vi "Open Form.vi"(8 "error in (no error)":errorcluster, 9 "Caller Name":T1, 10 "Form Config":refnum<class "Form Model Configuration.lvclass">, 11 "Form Server in":refnum<class "Form Server.lvclass">) -> (0 "error out":errorcluster, 3 "Form Server out":refnum<class "Form Server.lvclass">)   [LabVIEW 2020, in "Form Server.lvlib" / "Form Server.lvclass"]
uses:
  Form Server.lvclass
  C:/Program Files (x86)/National Instruments/LabVIEW 2020/vi.lib/ActorFramework/Actor/Actor.lvclass
  Forms Model/Form Model Configuration/Form Model Configuration Class/Form Model Configuration.lvclass
  Autoclose manager/Form ID.ctl
  Form Server.lvclass/Form Server.ctl
  Form Server Configuration/Form Server Configuration.lvclass/Form Server Configuration.ctl
  Forms Model/Form Model Actor/Form Model.lvclass
  Autoclose manager/Open Close Logic.lvclass
  <vilib>/ActorFramework/Actor/Actor.lvclass
  Form Server Configuration/Form Server Configuration.lvclass
  Form Server Interfaces.lvlib
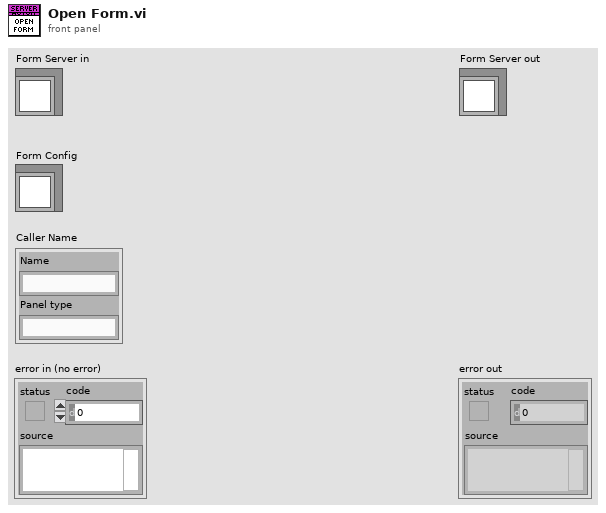
[diagram p1: front panel]
types:
  T1 = typedef "Form Server Interfaces.lvlib/Form ID.ctl" = cluster{"Name":string, "Panel type":string}
  T2 = map{T1, refnum<class "Message Enqueuer.lvclass">}
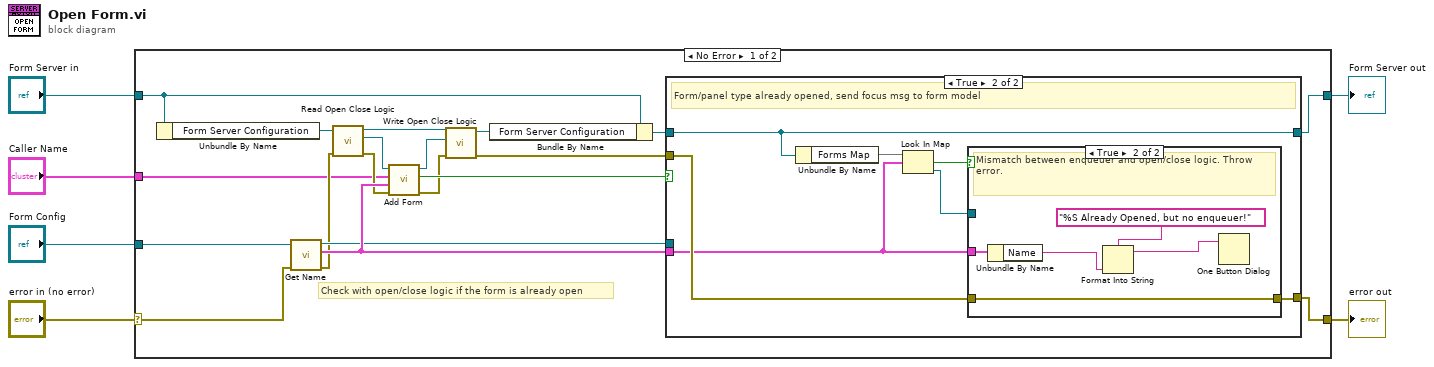
[diagram p0: block diagram]
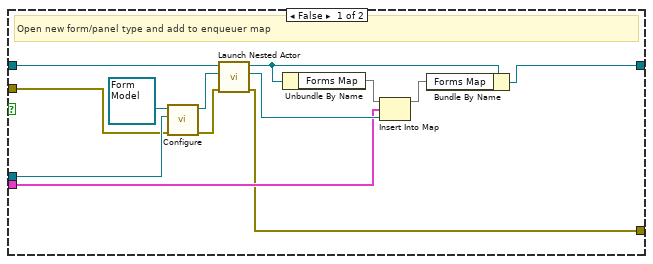
[diagram p2: hidden frame]
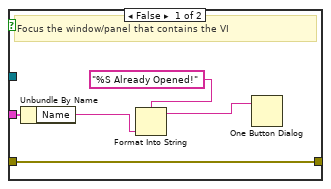
[diagram p3: hidden frame]
diagram:
  n1 = case shown="No Error" "error in (no error)" {
    selector: "error in (no error)" -> [w15 w57]
    tunnel: [w8 w57] -> w5
    tunnel: [w10 w56] -> w3
    tunnel: "Form Server in" -> [w20 w56]
    tunnel: "Form Config" -> [w25 _]
    tunnel: "Caller Name" -> [w7 _]
    frame No Error {
      # "Check with open/close logic if the form is already open"
      n2 = Unbundle By Name(w20) -> ("Form Server Configuration"=w24:refnum<class "Form Server Configuration.lvclass">)
      n3 = call-dynamic "Get Name.vi"("error in (no error)"=w15, "Form Configuration in"=w25) -> ("error out"=w14:errorcluster, "Form ID"=w17:T1, "Form Configuration out"=w16:refnum<class "Form Model Configuration.lvclass">)  [unwired: 7 in]
      n4 = call "Read Open Close Logic.vi"("error in (no error)"=w14, "Form Server Configuration in"=w24) -> ("error out"=w13:errorcluster, "Form Server Interfaces.lvlib:Open Close Logic.lvclass"=w23:refnum<class "Open Close Logic.lvclass">, "Form Server Configuration out"=w21:refnum<class "Form Server Configuration.lvclass">)  [unwired: 7 in]
      n5 = call-dynamic "Add Form.vi"("error in (no error)"=w13, "Nested"=w17, "Caller"=w7, "Autoclose manager in"=w23) -> ("error out"=w12:errorcluster, "Already opened?"=w18:bool, "Autoclose manager out"=w22:refnum<class "Open Close Logic.lvclass">)  [unwired: 5 in]
      n6 = call "Write Open Close Logic.vi"("error in (no error)"=w12, "Form Server Interfaces.lvlib:Open Close Logic.lvclass"=w22, "Form Server Configuration in"=w21) -> ("error out"=w9:errorcluster, "Form Server Configuration out"=w19:refnum<class "Form Server Configuration.lvclass">)  [unwired: 7 in]
      n7 = Bundle By Name(cluster=w20, "Form Server Configuration"=w19) -> (w11:refnum<class "Form Server.lvclass">)
      n8 = case shown="True" w18 {
        tunnel: w17 -> [w29 w39]
        tunnel: w16 -> [w32 _]
        tunnel: w11 -> [w31 w45]
        tunnel: [w30 w45] -> w10
        tunnel: w9 -> [w28 w41]
        tunnel: [w26 w40] -> w8
        frame False {
          # "Open new form/panel type and add to enqueuer map"
          n9 = call "Configure.vi"("error in (no error)"=w28, "Configuration"=w32, "Form Model in"=refnum<class "Form Model.lvclass"> refnum ("Form Model.lvlib:Form Model.lvclass")) -> ("error out"=w27:errorcluster, "Form Model out"=w34:refnum<class "Form Model.lvclass">)  [unwired: 7 in]
          n10 = call <vilib>:"Launch Nested Actor.vi"("error in (no error)"=w27, "Nested Actor"=w34, "Caller Actor in"=w31) -> ("error out"=w26:errorcluster, "Nested Actor's Enqueuer"=w38:refnum<class "Message Enqueuer.lvclass">, "Caller Actor out"=w36:refnum<class "Form Server.lvclass">)  [unwired: 6 in]
          n11 = Unbundle By Name(w36) -> ("Forms Map"=w35:T2)
          n12 = Insert Into Map(map in=w35, key=w29, value=w38) -> (map out=w37:T2)  [unwired: 2 out]
          n13 = Bundle By Name(cluster=w36, "Forms Map"=w37) -> (w30:refnum<class "Form Server.lvclass">)
        }
        frame True {
          # "Form/panel type already opened, send focus msg to form model"
          n14 = Unbundle By Name(w45) -> ("Forms Map"=w44:T2)
          n15 = Look In Map(map=w44, key=w39) -> (key not found?=w43:bool, value=w42:refnum<class "Message Enqueuer.lvclass">)  [unwired: 1 in]
          n16 = case shown="True" w43 {
            tunnel: w42 -> [_ _]
            tunnel: w41 -> [w50 w55]
            tunnel: [w50 w55] -> w40
            tunnel: w39 -> [w49 w51]
            frame False {
              # "Focus the window/panel that contains the VI"
              n17 = Unbundle By Name(w49) -> ("Name"=w47:string)
              n18 = Format Into String(format string="%S Already Opened!", w47) -> (resulting string=w46:string)  [unwired: 2 in, 1 out]
              n19 = One Button Dialog(message=w46) -> ()  [unwired: 1 in, 1 out]
            }
            frame True {
              # "Mismatch between enqueuer and open/close logic. Throw error."
              n20 = Unbundle By Name(w51) -> ("Name"=w53:string)
              n21 = Format Into String(format string="%S Already Opened, but no enqueuer!", w53) -> (resulting string=w54:string)  [unwired: 2 in, 1 out]
              n22 = One Button Dialog(message=w54) -> ()  [unwired: 1 in, 1 out]
            }
          }
        }
      }
    }
    frame Error {
    }
  }
  "error out" <- w5
  "Form Server out" <- w3
